vi "BestYInversoV1.vi"(8 "Field defense":dbl[](array[numeric]), 9 "atacando contra":bool, 10 "IA State":T1={"our_robots"=[], "enemy_robots"=[], "balls"=[], "geometry"={"line_width"=0, "field_length"=0, "field_width"=0, "boundary_width"=0, "referee_width"=0, "goal_width"=0, "goal_depth"=0, "goal_wall_width"=0, "center_circle_radius"=0, "defense_radius"=0, "defense_stretch"=0, "free_kick_from_defense_dist"=0, "penalty_spot_from_field_line_dist"=0, "penalty_line_from_spot_dist"=0}, "IA Judge"={"stage"="", "command"="", "our_goalie_id"=0.0, "enemy_goalie_id"=0.0, "command enum"=enum."Halt", "Time"=enum."Azul"}, "Received Timestamp"=timestamp(0 s since 1904-01-01), "Events"={"Touch"=FALSE, "Ball out"=FALSE, "id touch"=0.0, "Ball out of \nVision"=FALSE, "Ball inside \nGoalie area"=FALSE, "Robot not responding"=FALSE, "Robots responding status"=[1.0, 1.0, 1.0, 1.0, 1.0, 1.0], "Enemy Ball \nPossession"=FALSE, "Pass State"=FALSE, "id end of pass"=0.0, "Kick"=FALSE, "Id ini Possession"=0.0, "Ball Possesion"=FALSE, "Id Possesion"=0.0, "Direct Kick"=FALSE, "2nd Strk Ativo"=FALSE}}) -> (1 "Position":dbl[](array[numeric]))   [LabVIEW 2017]
uses:
  Core/AI Input.ctl
  Core/AI Robot.ctl
  Intel/Functions Enum.ctl
  Intel/AttackerStates.ctl
  Path Planning/RRT/PathDests.ctl
  Path Planning/RRT/PathDest.ctl
  Core/AI Ball.ctl
  Core/Field Size.ctl
  Core/AI Judge.ctl
  Intel/Command Enum.ctl
  Events/Events.ctl
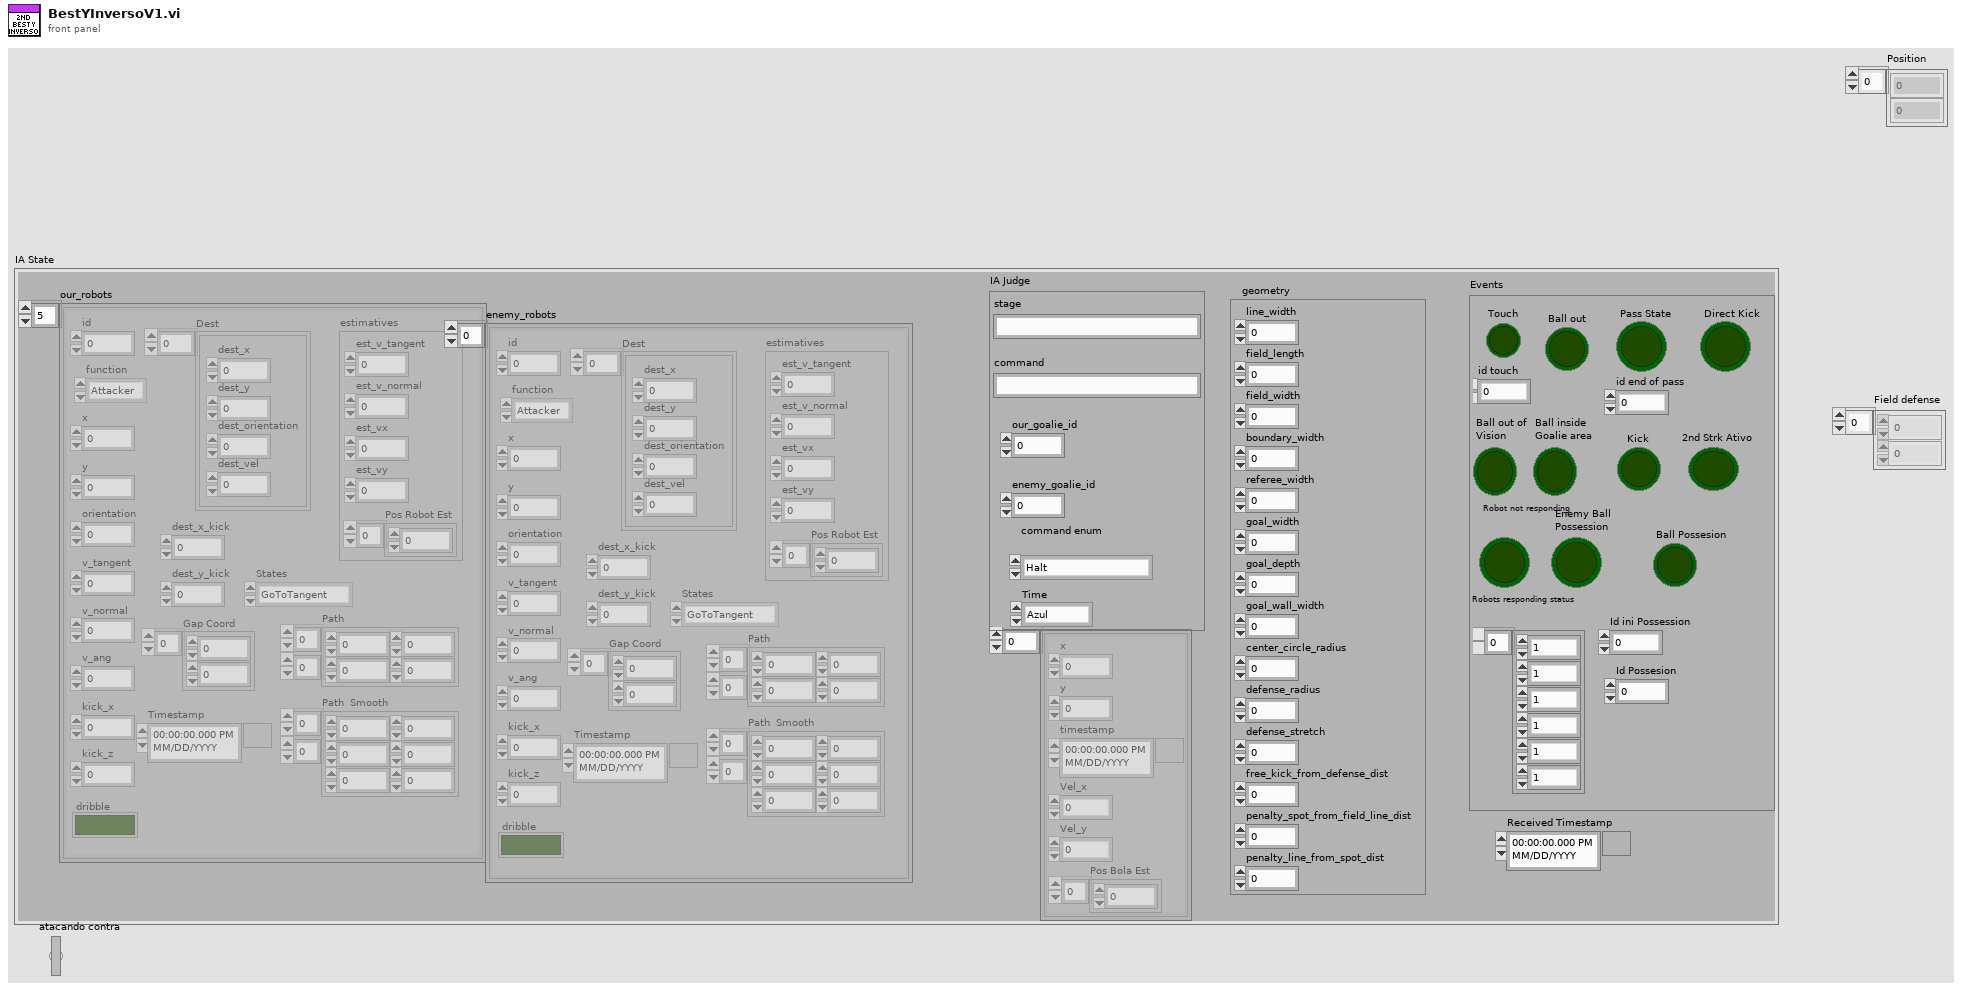
[diagram p1: front panel]
types:
  T1 = typedef "AI Input.ctl" = cluster{"our_robots":T2[], "enemy_robots":T2[], "balls":T7[], "geometry":T8, "IA Judge":T9, "Received Timestamp":timestamp, "Events":T11}
  T2 = typedef "AI Robot.ctl" = cluster{"id":u32, "function":T3, "x":dbl, "y":dbl, "orientation":dbl, "v_tangent":dbl, "v_normal":dbl, "v_ang":dbl, "kick_x":dbl, "kick_z":dbl, "dribble":bool, "Timestamp":timestamp, "estimatives":cluster{"est_v_tangent":dbl, "est_v_normal":dbl, "est_vx":dbl, "est_vy":dbl, "Pos Robot Est":dbl[]}, "dest_x_kick":dbl, "dest_y_kick":dbl, "Gap Coord":dbl[], "States":T4, "Path ":dbl[][], "Path  Smooth":dbl[][], "Dest":T5}
  T3 = typedef "Functions Enum.ctl" = enum16{"2nd Striker", "Attacker", "Goalie", "Defender", "Striker", "Goto 0", "Dummy", "Kicker", "ZigZag 0", "ZigZag 1", "ZigZag 2", "ZigZag 3", "ZigZag 4", "ZigZag 5", "ZigZag 6", "ZigZag 7", "ZigZag 8", ""}
  T4 = typedef "AttackerStates.ctl" = enum16{"Pass", "GoToTangent", "BallGetting", "GoToKick", ""}
  T5 = typedef "PathDests.ctl" = T6[]
  T6 = typedef "PathDest.ctl" = cluster{"dest_x":dbl, "dest_y":dbl, "dest_orientation":dbl, "dest_vel":dbl}
  T7 = typedef "AI Ball.ctl" = cluster{"x":dbl, "y":dbl, "timestamp":timestamp, "Vel_x":dbl, "Vel_y":dbl, "Pos Bola Est":dbl[]}
  T8 = typedef "Field Size.ctl" = cluster{"line_width":u32, "field_length":u32, "field_width":u32, "boundary_width":u32, "referee_width":u32, "goal_width":u32, "goal_depth":u32, "goal_wall_width":u32, "center_circle_radius":u32, "defense_radius":u32, "defense_stretch":u32, "free_kick_from_defense_dist":u32, "penalty_spot_from_field_line_dist":u32, "penalty_line_from_spot_dist":u32}
  T9 = typedef "AI Judge.ctl" = cluster{"stage":string, "command":string, "our_goalie_id":dbl, "enemy_goalie_id":dbl, "command enum":T10, "Time":enum16{"Azul", "Amarelo"}}
  T10 = typedef "Command Enum.ctl" = enum16{"Halt", "Stop", "Force Start", "PKA Normal Start", "Prepare Kickoff Ally", "PKE Normal Start", "Prepare Kickoff Enemy", "Prepare Penalty Ally", "PPA Normal Start", "Prepare Penalty Enemy", "PPE Normal Start", "Direct Free Enemy", "Direct Free Ally", "Indirect Free Enemy", "Indirect Free Ally", "Timeout Enemy", "Timeout Ally", "Goal Enemy", "Goal Ally", "Ball Placement Enemy", "Ball Placement Ally", "Normal Half Time", "Extra Time Break", "Extra Half Time", "None", "Post Game"}
  T11 = typedef "Events.ctl" = cluster{"Touch":bool, "Ball out":bool, "id touch":dbl, "Ball out of \nVision":bool, "Ball inside \nGoalie area":bool, "Robot not responding":bool, "Robots responding status":dbl[], "Enemy Ball \nPossession":bool, "Pass State":bool, "id end of pass":dbl, "Kick":bool, "Id ini Possession":dbl, "Ball Possesion":bool, "Id Possesion":dbl, "Direct Kick":bool, "2nd Strk Ativo":bool}
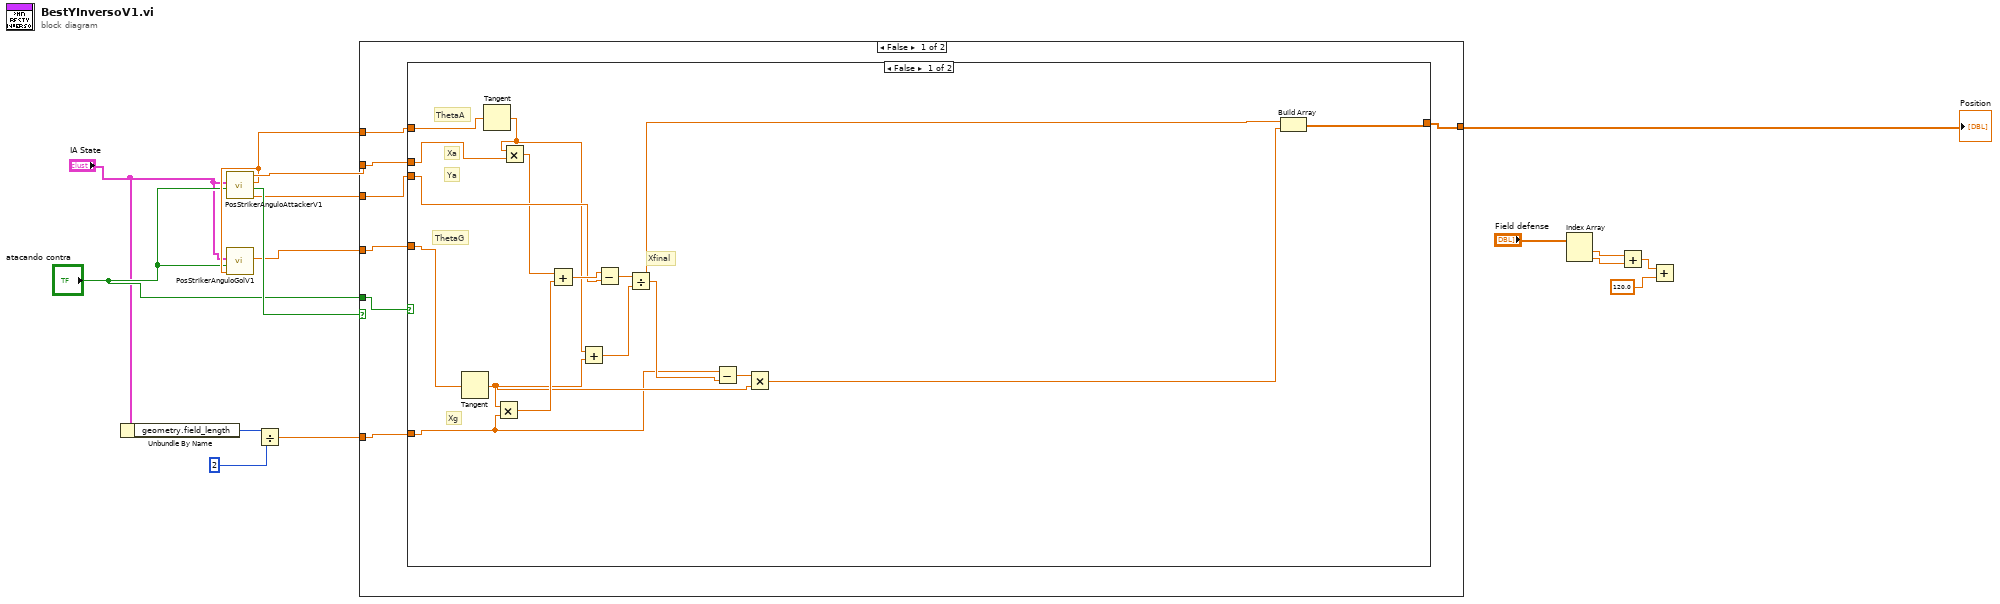
[diagram p0: block diagram]
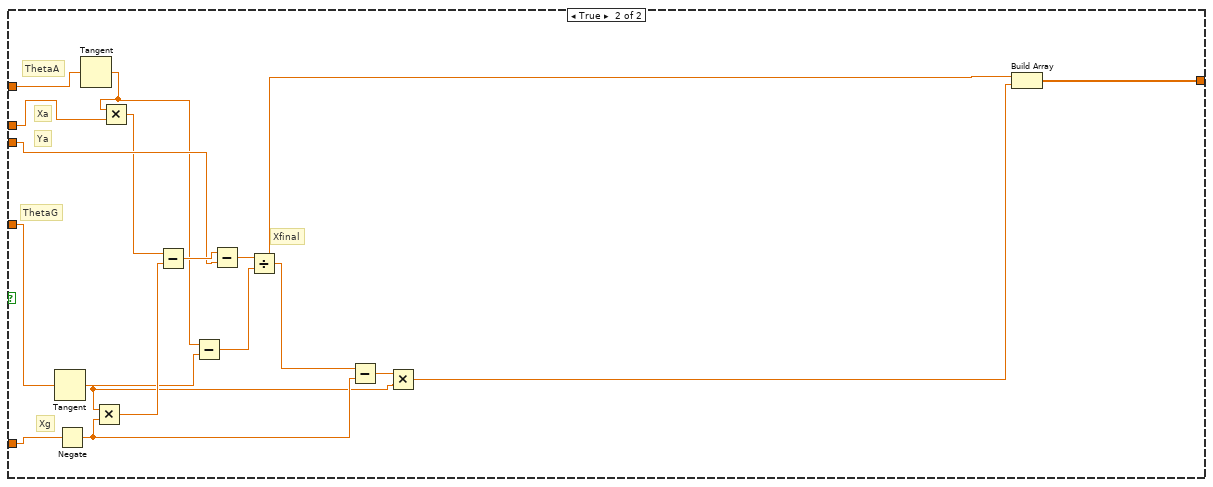
[diagram p2: hidden frame]
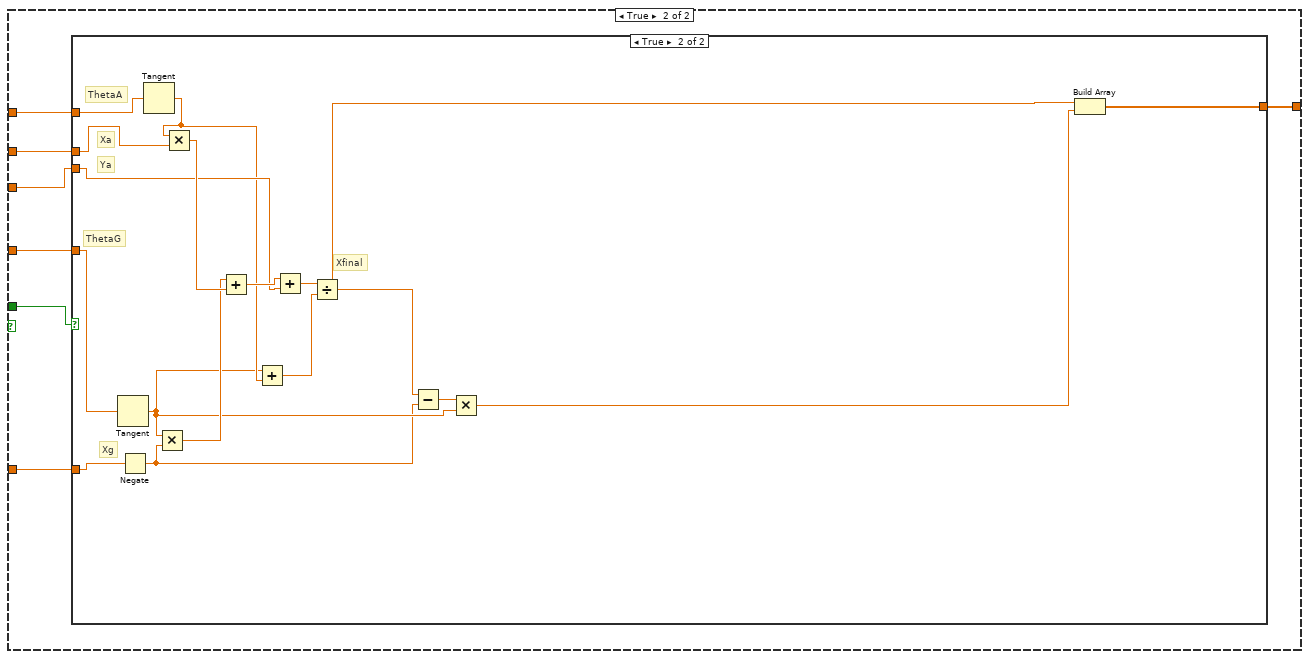
[diagram p3: hidden frame]
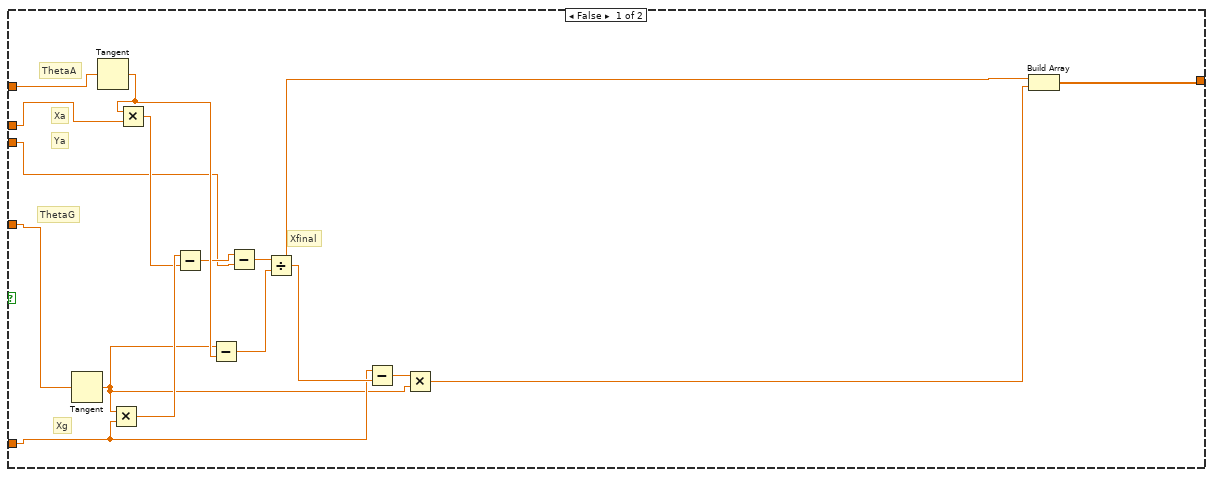
[diagram p4: hidden frame]
diagram:
  n1 = Unbundle By Name("IA State") -> ("geometry.field_length"=w16:u32)
  n2 = call "PosStrikerAnguloAttackerV1.vi"("atacando contra"="atacando contra", "IA State"="IA State") -> ("YdoAttacker 2"=w5:dbl, "AttackerPositive?"=w6:bool, "theta final"=w4:dbl, "XdoAttacker 2"=w7:dbl)  [unwired: 6 in]
  n3 = call "PosStrikerAnguloGolV1.vi"("AnguloAttacker"=w4, "atacando contra"="atacando contra", "IA State"="IA State") -> ("theta final"=w2:dbl)  [unwired: 8 in]
  n4 = Divide(x=w16, y=u32 2) -> (x/y=w14:dbl)
  n5 = case shown="False" w6 {
    tunnel: "atacando contra" -> [w17 w63]
    tunnel: w4 -> [w22 w62]
    tunnel: w7 -> [w21 w61]
    tunnel: w5 -> [w20 w60]
    tunnel: w2 -> [w19 w59]
    tunnel: w14 -> [w18 w58]
    tunnel: [w23 w57] -> w13
    frame False {
      n6 = case shown="False" w17 {
        tunnel: w22 -> [w33 w53]
        tunnel: w21 -> [w32 w54]
        tunnel: w20 -> [w31 w51]
        tunnel: w19 -> [w34 w55]
        tunnel: w18 -> [w24 w56]
        tunnel: [w30 w46] -> w23
        frame False {
          # "Xfinal"
          # "Xg"
          # "ThetaG"
          # "Ya"
          # "Xa"
          # "ThetaA"
          n7 = Tangent(1:w34) -> (0:w26:dbl)
          n8 = Tangent(1:w33) -> (0:w27:dbl)
          n9 = Multiply(x=w26, y=w24) -> (x*y=w29:dbl)
          n10 = Multiply(x=w27, y=w32) -> (x*y=w28:dbl)
          n11 = Add(x=w28, y=w29) -> (x+y=w35:dbl)
          n12 = Add(x=w27, y=w26) -> (x+y=w37:dbl)
          n13 = Subtract(x=w35, y=w31) -> (x-y=w36:dbl)
          n14 = Divide(x=w36, y=w37) -> (x/y=w25:dbl)
          n15 = Subtract(x=w24, y=w25) -> (x-y=w38:dbl)
          n16 = Multiply(x=w38, y=w26) -> (x*y=w39:dbl)
          n17 = Build Array(w25, w39) -> (w30:dbl[])
        }
        frame True {
          # "Xfinal"
          # "Xg"
          # "ThetaG"
          # "Ya"
          # "Xa"
          # "ThetaA"
          n18 = Tangent(1:w55) -> (0:w40:dbl)
          n19 = Negate(x=w56) -> (-x=w45:dbl)
          n20 = Tangent(1:w53) -> (0:w41:dbl)
          n21 = Multiply(x=w40, y=w45) -> (x*y=w43:dbl)
          n22 = Multiply(x=w41, y=w54) -> (x*y=w42:dbl)
          n23 = Subtract(x=w42, y=w43) -> (x-y=w52:dbl)
          n24 = Subtract(x=w41, y=w40) -> (x-y=w49:dbl)
          n25 = Subtract(x=w52, y=w51) -> (x-y=w50:dbl)
          n26 = Divide(x=w50, y=w49) -> (x/y=w44:dbl)
          n27 = Subtract(x=w44, y=w45) -> (x-y=w48:dbl)
          n28 = Multiply(x=w48, y=w40) -> (x*y=w47:dbl)
          n29 = Build Array(w44, w47) -> (w46:dbl[])
        }
      }
    }
    frame True {
      n30 = case shown="True" w63 {
        tunnel: w62 -> [w69 w93]
        tunnel: w61 -> [w68 w94]
        tunnel: w60 -> [w67 w89]
        tunnel: w59 -> [w70 w95]
        tunnel: w58 -> [w66 w96]
        tunnel: [w65 w84] -> w57
        frame False {
          # "Xfinal"
          # "Xg"
          # "ThetaG"
          # "Ya"
          # "Xa"
          # "ThetaA"
          n31 = Tangent(1:w70) -> (0:w64:dbl)
          n32 = Tangent(1:w69) -> (0:w78:dbl)
          n33 = Multiply(x=w64, y=w66) -> (x*y=w72:dbl)
          n34 = Multiply(x=w78, y=w68) -> (x*y=w71:dbl)
          n35 = Subtract(x=w72, y=w71) -> (x-y=w73:dbl)
          n36 = Subtract(x=w64, y=w78) -> (x-y=w75:dbl)
          n37 = Subtract(x=w73, y=w67) -> (x-y=w74:dbl)
          n38 = Divide(x=w74, y=w75) -> (x/y=w76:dbl)
          n39 = Subtract(x=w66, y=w76) -> (x-y=w77:dbl)
          n40 = Multiply(x=w77, y=w64) -> (x*y=w79:dbl)
          n41 = Build Array(w76, w79) -> (w65:dbl[])
        }
        frame True {
          # "Xfinal"
          # "Xg"
          # "ThetaG"
          # "Ya"
          # "Xa"
          # "ThetaA"
          n42 = Tangent(1:w95) -> (0:w82:dbl)
          n43 = Negate(x=w96) -> (-x=w81:dbl)
          n44 = Tangent(1:w93) -> (0:w83:dbl)
          n45 = Multiply(x=w82, y=w81) -> (x*y=w91:dbl)
          n46 = Multiply(x=w83, y=w94) -> (x*y=w92:dbl)
          n47 = Add(x=w91, y=w92) -> (x+y=w90:dbl)
          n48 = Add(x=w82, y=w83) -> (x+y=w87:dbl)
          n49 = Add(x=w90, y=w89) -> (x+y=w88:dbl)
          n50 = Divide(x=w88, y=w87) -> (x/y=w80:dbl)
          n51 = Subtract(x=w80, y=w81) -> (x-y=w86:dbl)
          n52 = Multiply(x=w86, y=w82) -> (x*y=w85:dbl)
          n53 = Build Array(w80, w85) -> (w84:dbl[])
        }
      }
    }
  }
  "Position" <- w13
  n54 = Index Array(array="Field defense") -> (element #1=w11:dbl, element #2=w10:dbl)  [unwired: 2 in]
  n55 = Add(x=w11, y=w10) -> (x+y=w9:dbl)
  n56 = Add(x=w9, y=120.0) -> ()  [unwired: 1 out]
